vi "OP3_RODAGGIO.vi"(0 "Esito 2 in":cluster{"Si":bool, "No":bool}, 1 "Esito 3 in":cluster{"Si":bool, "No":bool}, 2 "Esito 4 in":cluster{"Si":bool, "No":bool}, 3 "Esito 5 in":cluster{"Si":bool, "No":bool}, 4 "Esito 6 in":cluster{"Si":bool, "No":bool}, 5 "Esito 7 in":cluster{"Si":bool, "No":bool}, 6 "Esito 8 in":cluster{"Si":bool, "No":bool}, 7 "Esito 9 in":cluster{"Si":bool, "No":bool}, 8 "Esito 1 in":cluster{"Si":bool, "No":bool}, 9 "Tasto premuto":T1(array[ring]), 10 "Tipo specifica":string, 12 "Stato in":u16, 14 "Stato out":u16) -> (16 "Dato":string[](array[string]), 17 "ANNULLA PROVA":bool, 18 "Esito 1 out":T2, 19 "i out":i32=1, 20 "Esito 2 out":T2, 21 "Esito 3 out":T2, 22 "Esito 4 out":T2, 23 "Esito 5 out":T2, 24 "Esito 6 out":T2, 25 "Esito 7 out":T2, 26 "Esito 8 out":T2, 27 "Esito 9 out":T2)   [LabVIEW 2022 SP3]
uses:
  Labview/Globali.vi
panel:
  in  "i max":i32
  in  "i":i32=1
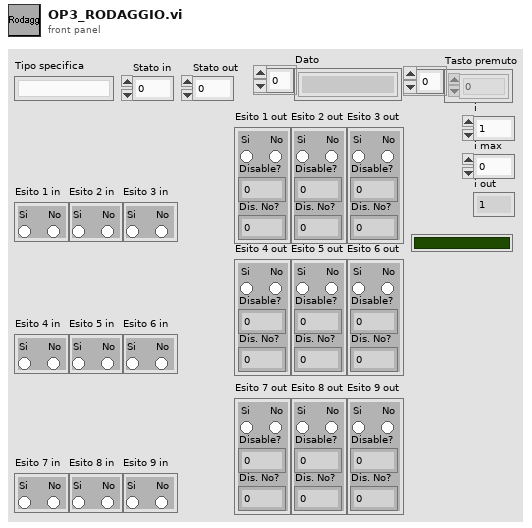
[diagram p1: front panel]
types:
  T1 = enum16{"0", "1", "2", "3", "4", "5", "6", "7", "8", "9", "A", "B", "C", "D", "E", "F", "G", "H", "I", "J", "K", "L", "M", "N", "O", "P", "Q", "R", "S", "T", "U", "V", "W", "X", "Y", "Z", "F1", "F2", "F3", "F4", "F5", "F6", "F7", "F8", "F9", "F10", "F11", "F12", "F13", "F14", "F15", "ADD", "BACK", "BACKSLASH", "CAPITAL", "COMMA", "DECIMAL", "DELETE", "DIVIDE", "DOWN", "END", "EQUALS", "ESCAPE", "GRAVE (`)", "HOME", "INSERT", "LBRACKET", "LCONTROL", "LEFT", "L ALT", "LSHIFT", "LWIN", "MINUS", "MULTIPLY", "NEXT", "NUMLOCK", "NUMPAD_0", "NUMPAD_1", "NUMPAD_2", "NUMPAD_3", "NUMPAD_4", "NUMPAD_5", "NUMPAD_6", "NUMPAD_7", "NUMPAD_8", "NUMPAD_9", "PAUSE", "PERIOD", "PRIOR (PG UP)", "RBRACKET", "RCONTROL", "RETURN", "RIGHT", "R ALT", "RSHIFT", "RWIN", "SCROLL", "SEMICOLON", "SLASH", "SPACE", "SUBTRACT", "TAB", "UP", "ENTER (num pad)", "' (quote)"}[]
  T2 = cluster{"Disable?":i16, "Si":bool, "No":bool, "Dis. No?":i16}
  T3 = cluster{"Esito 1 out":cluster{"Disable?":i16, "Si":bool, "No":bool, "Dis. No?":i16}, "Esito 2 out":cluster{"Disable?":i16, "Si":bool, "No":bool, "Dis. No?":i16}, "Esito 3 out":cluster{"Disable?":i16, "Si":bool, "No":bool, "Dis. No?":i16}, "Esito 4 out":cluster{"Disable?":i16, "Si":bool, "No":bool, "Dis. No?":i16}, "Esito 5 out":cluster{"Disable?":i16, "Si":bool, "No":bool, "Dis. No?":i16}, "Esito 6 out":cluster{"Disable?":i16, "Si":bool, "No":bool, "Dis. No?":i16}, "Esito 7 out":cluster{"Disable?":i16, "Si":bool, "No":bool, "Dis. No?":i16}, "Esito 8 out":cluster{"Disable?":i16, "Si":bool, "No":bool, "Dis. No?":i16}, "Esito 9 out":cluster{"Disable?":i16, "Si":bool, "No":bool, "Dis. No?":i16}}
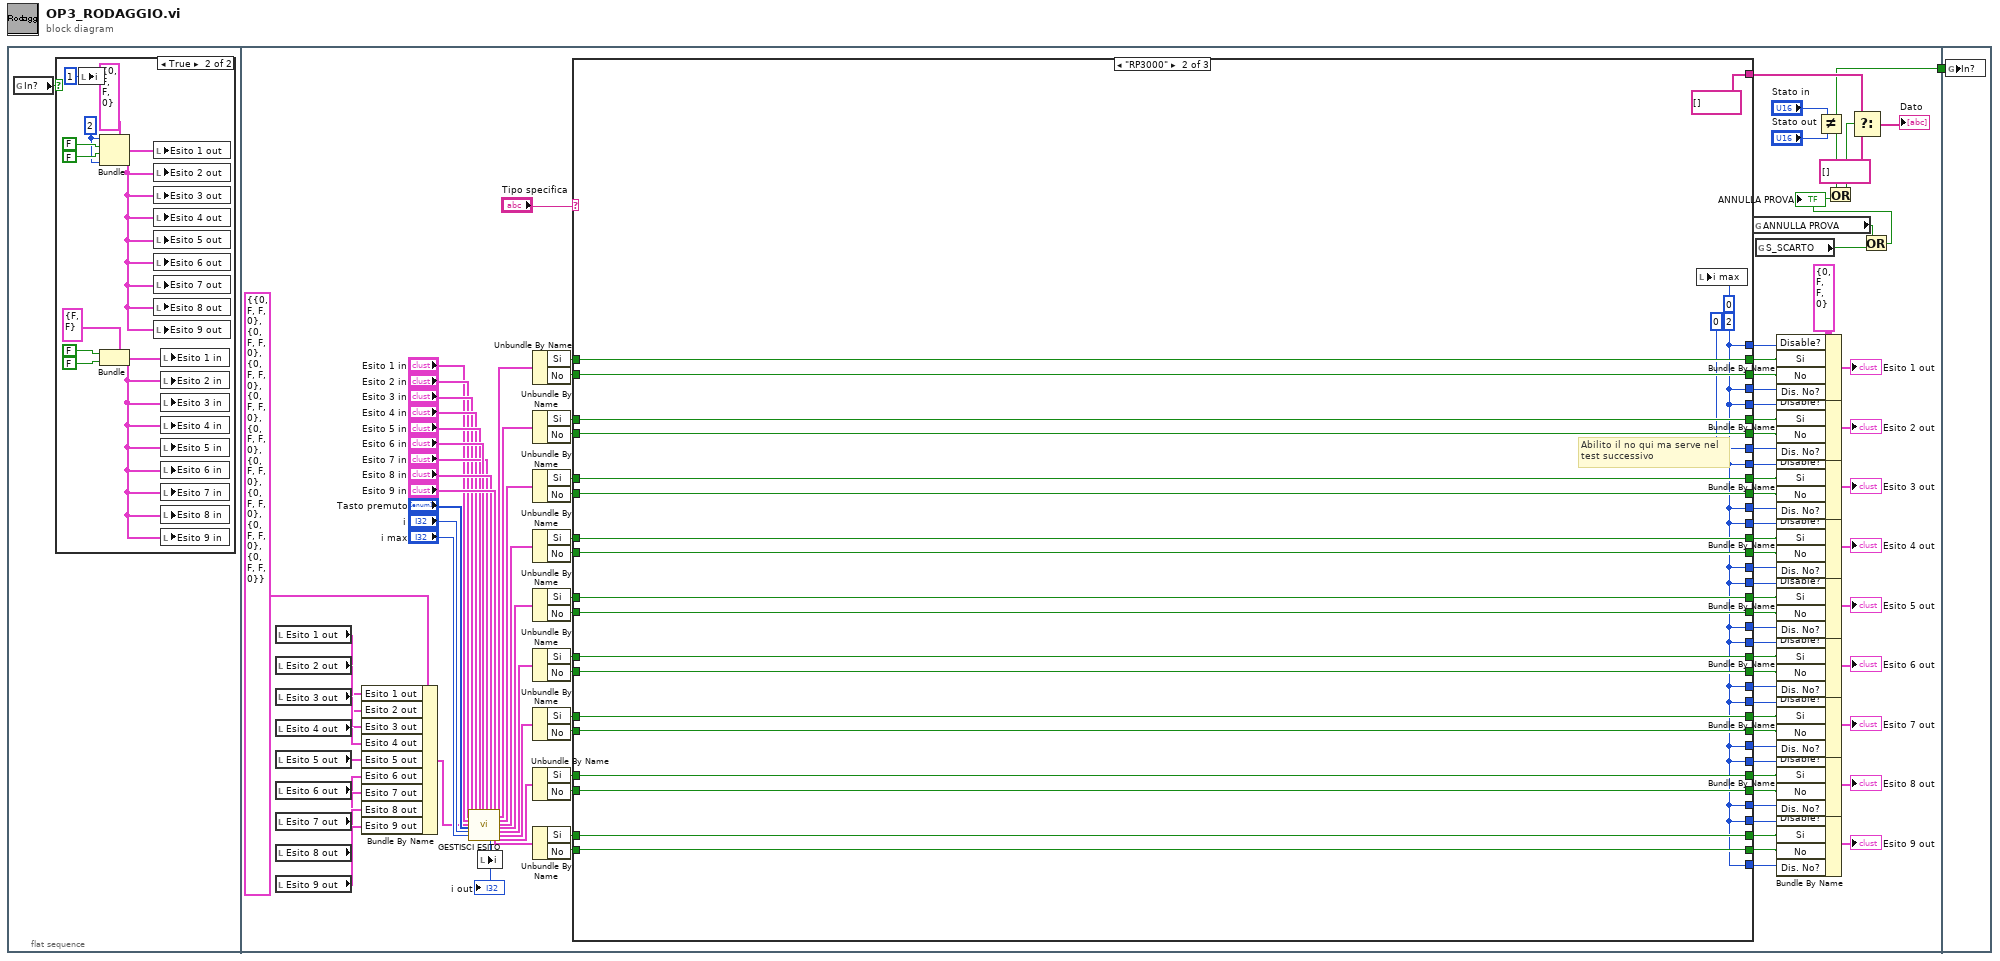
[diagram p0: block diagram]
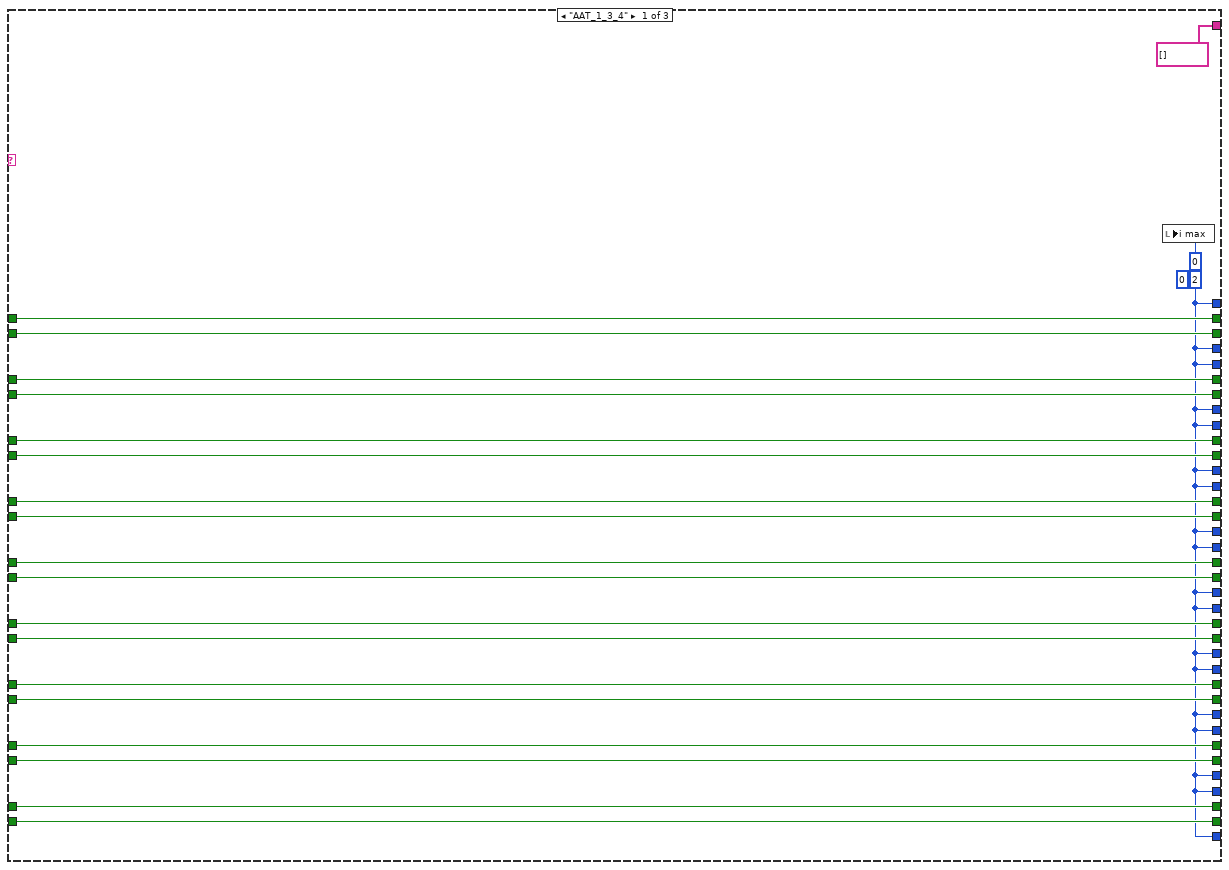
[diagram p3: hidden frame]
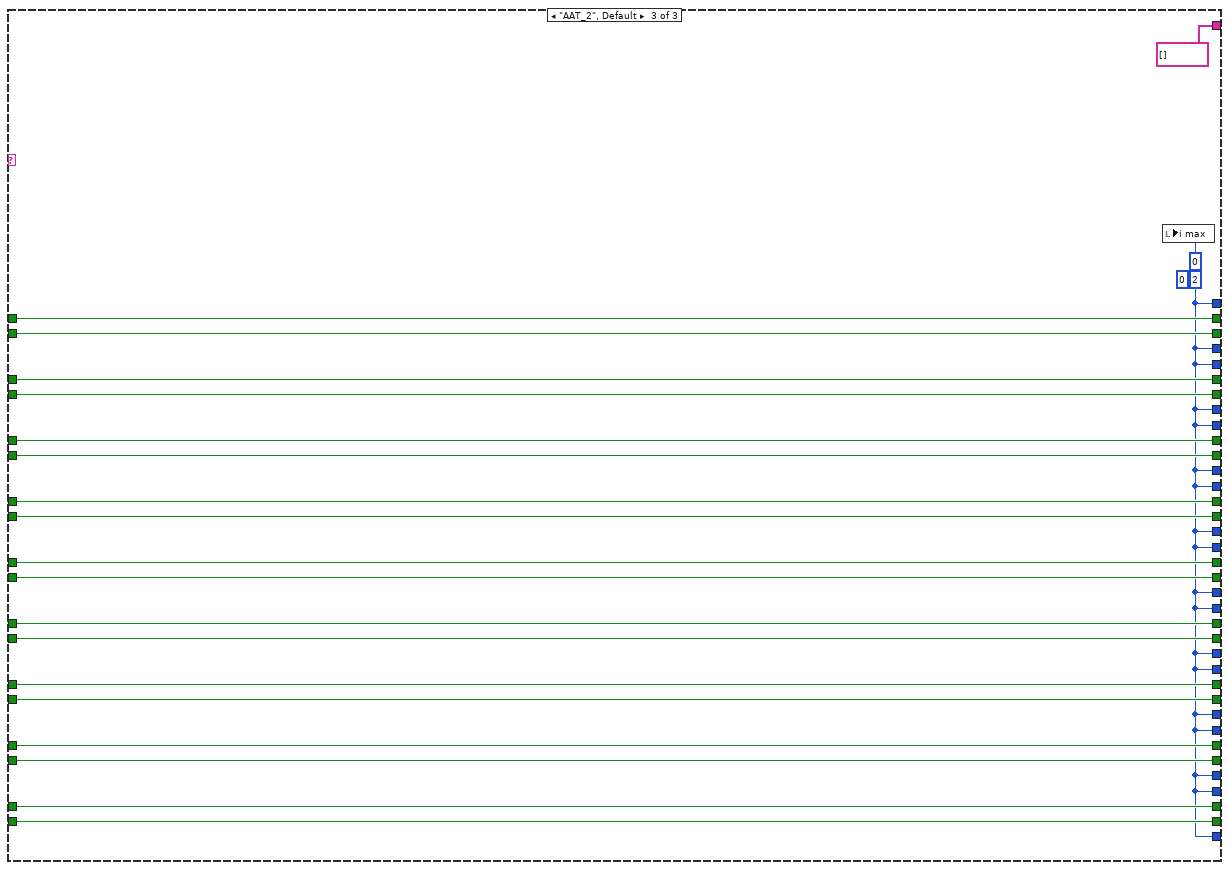
[diagram p4: hidden frame]
diagram:
  n1 = flat-sequence {
    tunnel: [w17] -> w1
    tunnel: w1 -> [w185]
    frame #0 {
      n2 = global read "Globali.vi" "In?"() -> (w2:bool)
      n3 = case shown="True" w2 {
        frame False {
        }
        frame True {
          w9 = i16 2 ("Disable?")
          n4 = local write "i"(1 ("i")) -> ()
          n5 = Bundle(cluster=T2 {"Disable?"=0, "Si"=FALSE, "No"=FALSE, "Dis. No?"=0} ("Esito 1 out"), "Disable?"=w9, "Si"=FALSE, "No"=FALSE, "Dis. No?"=w9) -> (w8:T2)
          n6 = Bundle(cluster=cluster{"Si":bool, "No":bool} {"Si"=FALSE, "No"=FALSE} ("Esito 1 in"), "Si"=FALSE, "No"=FALSE) -> (w6:cluster{"Si":bool, "No":bool})
          n7 = local write "Esito 1 out"(w8) -> ()
          n8 = local write "Esito 2 out"(w8) -> ()
          n9 = local write "Esito 3 out"(w8) -> ()
          n10 = local write "Esito 4 out"(w8) -> ()
          n11 = local write "Esito 5 out"(w8) -> ()
          n12 = local write "Esito 6 out"(w8) -> ()
          n13 = local write "Esito 7 out"(w8) -> ()
          n14 = local write "Esito 8 out"(w8) -> ()
          n15 = local write "Esito 9 out"(w8) -> ()
          n16 = local write "Esito 1 in"(w6) -> ()
          n17 = local write "Esito 2 in"(w6) -> ()
          n18 = local write "Esito 3 in"(w6) -> ()
          n19 = local write "Esito 4 in"(w6) -> ()
          n20 = local write "Esito 5 in"(w6) -> ()
          n21 = local write "Esito 6 in"(w6) -> ()
          n22 = local write "Esito 7 in"(w6) -> ()
          n23 = local write "Esito 8 in"(w6) -> ()
          n24 = local write "Esito 9 in"(w6) -> ()
        }
      }
    }
    frame #1 {
      w60 = T2 {"Disable?"=0, "Si"=FALSE, "No"=FALSE, "Dis. No?"=0} ("Esito 1 out")
      n25 = local read "Esito 1 out"() -> (w38:T2)
      n26 = local read "Esito 2 out"() -> (w39:T2)
      n27 = local read "Esito 3 out"() -> (w40:T2)
      n28 = local read "Esito 4 out"() -> (w41:T2)
      n29 = local read "Esito 5 out"() -> (w42:T2)
      n30 = local read "Esito 6 out"() -> (w43:T2)
      n31 = local read "Esito 7 out"() -> (w44:T2)
      n32 = local read "Esito 8 out"() -> (w45:T2)
      n33 = local read "Esito 9 out"() -> (w46:T2)
      n34 = Bundle By Name(cluster=T3 {"Esito 1 out"={"Disable?"=0, "Si"=FALSE, "No"=FALSE, "Dis. No?"=0}, "Esito 2 out"={"Disable?"=0, "Si"=FALSE, "No"=FALSE, "Dis. No?"=0}, "Esito 3 out"={"Disable?"=0, "Si"=FALSE, "No"=FALSE, "Dis. No?"=0}, "Esito 4 out"={"Disable?"=0, "Si"=FALSE, "No"=FALSE, "Dis. No?"=0}, "Esito 5 out"={"Disable?"=0, "Si"=FALSE, "No"=FALSE, "Dis. No?"=0}, "Esito 6 out"={"Disable?"=0, "Si"=FALSE, "No"=FALSE, "Dis. No?"=0}, "Esito 7 out"={"Disable?"=0, "Si"=FALSE, "No"=FALSE, "Dis. No?"=0}, "Esito 8 out"={"Disable?"=0, "Si"=FALSE, "No"=FALSE, "Dis. No?"=0}, "Esito 9 out"={"Disable?"=0, "Si"=FALSE, "No"=FALSE, "Dis. No?"=0}} ("Cluster"), "Esito 1 out"=w38, "Esito 2 out"=w39, "Esito 3 out"=w40, "Esito 4 out"=w41, "Esito 5 out"=w42, "Esito 6 out"=w43, "Esito 7 out"=w44, "Esito 8 out"=w45, "Esito 9 out"=w46) -> (w47:T3)
      n35 = call "GESTISCI ESITO.vi"("Esito 3 in"="Esito 3 in", "Esito 2 in"="Esito 2 in", "Esito 1 in"="Esito 1 in", "Cluster"=w47, "Tasto premuto"="Tasto premuto", "i in"="i", "i max"="i max", "Esito 4 in"="Esito 4 in", "Esito 5 in"="Esito 5 in", "Esito 6 in"="Esito 6 in", "Esito 7 in"="Esito 7 in", "Esito 8 in"="Esito 8 in", "Esito 9 in"="Esito 9 in") -> ("i out"=w18:i32, "Esito 9 in 2"=w36:cluster{"Si":bool, "No":bool}, "Esito 1 in 2"=w28:cluster{"Si":bool, "No":bool}, "Esito 2 in 2"=w29:cluster{"Si":bool, "No":bool}, "Esito 3 in 2"=w30:cluster{"Si":bool, "No":bool}, "Esito 4 in 2"=w31:cluster{"Si":bool, "No":bool}, "Esito 5 in 2"=w32:cluster{"Si":bool, "No":bool}, "Esito 6 in 2"=w33:cluster{"Si":bool, "No":bool}, "Esito 7 in 2"=w34:cluster{"Si":bool, "No":bool}, "Esito 8 in 2"=w35:cluster{"Si":bool, "No":bool})  [unwired: 5 in]
      "i out" <- w18
      n36 = local write "i"(w18) -> ()
      n37 = Unbundle By Name(w28) -> ("Si"=w84:bool, "No"=w83:bool)
      n38 = Unbundle By Name(w29) -> ("Si"=w67:bool, "No"=w68:bool)
      n39 = Unbundle By Name(w30) -> ("Si"=w69:bool, "No"=w70:bool)
      n40 = Unbundle By Name(w31) -> ("Si"=w71:bool, "No"=w72:bool)
      n41 = Unbundle By Name(w32) -> ("Si"=w73:bool, "No"=w74:bool)
      n42 = Unbundle By Name(w33) -> ("Si"=w75:bool, "No"=w76:bool)
      n43 = Unbundle By Name(w34) -> ("Si"=w77:bool, "No"=w78:bool)
      n44 = Unbundle By Name(w35) -> ("Si"=w79:bool, "No"=w80:bool)
      n45 = Unbundle By Name(w36) -> ("Si"=w81:bool, "No"=w82:bool)
      n46 = case shown="\"RP3000\"" "Tipo specifica" {
        tunnel: [string[] [] ("Dato") string[] [] ("Dato") string[] [] ("Dato")] -> w64
        tunnel: [w123 w144 w166] -> w111
        tunnel: [w123 w144 w166] -> w110
        tunnel: [w123 w144 w166] -> w109
        tunnel: [w123 w144 w166] -> w108
        tunnel: [w123 w144 w166] -> w107
        tunnel: [w123 w144 w166] -> w106
        tunnel: [w123 w144 w166] -> w105
        tunnel: [w123 w144 w166] -> w104
        tunnel: [w123 w144 w166] -> w103
        tunnel: [w124 w146 w167] -> w102
        tunnel: [w131 w153 w174] -> w101
        tunnel: [w130 w152 w173] -> w100
        tunnel: [w132 w154 w175] -> w99
        tunnel: [w125 w147 w168] -> w98
        tunnel: [w141 w163 w184] -> w97
        tunnel: [w126 w148 w169] -> w96
        tunnel: [w140 w162 w183] -> w95
        tunnel: [w129 w151 w172] -> w94
        tunnel: [w139 w161 w182] -> w93
        tunnel: [w128 w150 w171] -> w92
        tunnel: [w138 w160 w181] -> w91
        tunnel: [w127 w149 w170] -> w90
        tunnel: [w137 w159 w180] -> w89
        tunnel: [w136 w158 w179] -> w88
        tunnel: [w135 w157 w178] -> w87
        tunnel: [w134 w156 w177] -> w86
        tunnel: [w133 w155 w176] -> w85
        tunnel: w84 -> [w124 w146 w167]
        tunnel: w83 -> [w131 w153 w174]
        tunnel: w82 -> [w133 w155 w176]
        tunnel: w81 -> [w134 w156 w177]
        tunnel: w80 -> [w135 w157 w178]
        tunnel: w79 -> [w136 w158 w179]
        tunnel: w78 -> [w137 w159 w180]
        tunnel: w77 -> [w127 w149 w170]
        tunnel: w76 -> [w138 w160 w181]
        tunnel: w75 -> [w128 w150 w171]
        tunnel: w74 -> [w139 w161 w182]
        tunnel: w73 -> [w129 w151 w172]
        tunnel: w72 -> [w140 w162 w183]
        tunnel: w71 -> [w126 w148 w169]
        tunnel: w70 -> [w141 w163 w184]
        tunnel: w69 -> [w125 w147 w168]
        tunnel: w68 -> [w132 w154 w175]
        tunnel: w67 -> [w130 w152 w173]
        tunnel: [w123 w144 w166] -> w59
        tunnel: [w123 0 w166] -> w58
        tunnel: [w123 w144 w166] -> w57
        tunnel: [w123 w144 w166] -> w56
        tunnel: [w123 w144 w166] -> w55
        tunnel: [w123 w144 w166] -> w54
        tunnel: [w123 w144 w166] -> w53
        tunnel: [w123 w144 w166] -> w52
        tunnel: [w123 w144 w166] -> w51
        frame "AAT_1_3_4" {
          w123 = 2
          (unwired) 0
          n47 = local write "i max"(0) -> ()
        }
        frame "RP3000" {
          w144 = 2
          # "Abilito il no qui ma serve nel\ntest successivo"
          n48 = local write "i max"(0) -> ()
        }
        frame "AAT_2", Default {
          w166 = 2
          (unwired) 0
          n49 = local write "i max"(0) -> ()
        }
      }
      n50 = global read "Globali.vi" "ANNULLA PROVA"() -> (w15:bool)
      n51 = global read "Globali.vi" "S_SCARTO"() -> (w14:bool)
      n52 = Bundle By Name(cluster=w60, "Disable?"=w111, "Si"=w102, "No"=w101, "Dis. No?"=w59) -> (→"Esito 1 out":T2)
      n53 = Bundle By Name(cluster=w60, "Disable?"=w110, "Si"=w100, "No"=w99, "Dis. No?"=w58) -> (→"Esito 2 out":T2)
      n54 = Bundle By Name(cluster=w60, "Disable?"=w109, "Si"=w98, "No"=w97, "Dis. No?"=w57) -> (→"Esito 3 out":T2)
      n55 = Bundle By Name(cluster=w60, "Disable?"=w108, "Si"=w96, "No"=w95, "Dis. No?"=w56) -> (→"Esito 4 out":T2)
      n56 = Bundle By Name(cluster=w60, "Disable?"=w107, "Si"=w94, "No"=w93, "Dis. No?"=w55) -> (→"Esito 5 out":T2)
      n57 = Bundle By Name(cluster=w60, "Disable?"=w106, "Si"=w92, "No"=w91, "Dis. No?"=w54) -> (→"Esito 6 out":T2)
      n58 = Bundle By Name(cluster=w60, "Disable?"=w105, "Si"=w90, "No"=w89, "Dis. No?"=w53) -> (→"Esito 7 out":T2)
      n59 = Bundle By Name(cluster=w60, "Disable?"=w104, "Si"=w88, "No"=w87, "Dis. No?"=w52) -> (→"Esito 8 out":T2)
      n60 = Bundle By Name(cluster=w60, "Disable?"=w103, "Si"=w86, "No"=w85, "Dis. No?"=w51) -> (→"Esito 9 out":T2)
      n61 = Not Equal?(x="Stato in", y="Stato out") -> (x != y?=w17:bool)
      n62 = Or(x=w15, y=w14) -> (x .or. y?=w13:bool)
      "ANNULLA PROVA" <- w13
      n63 = Or(x=w17, y=w13) -> (x .or. y?=w16:bool)
      n64 = Select(t=w64, s=w16, f=string[] [] ("Dato")) -> (s? t:f=→"Dato":string[])
    }
    frame #2 {
      n65 = global write "Globali.vi" "In?"(w185) -> ()
    }
  }
